vi "GenSignal.vi"(0 "Offset":dbl min=-1.0 max=1.0 step=0.1 format="%.2p", 1 "Reset Signal":bool, 2 "Formula":string="a*cos(w*t+p)", 4 "Amplitude":dbl=1.0 min=0.0 max=1.0 step=0.01 format="%.2f", 6 "Sampling Rate (MHz)":u32=1000, 7 "Phase":dbl format="%.2p", 8 "Start Time":dbl format="%#.6g", 9 "Duration (us)":dbl=1.0, 10 "Frequency (MHz)":dbl=200.0 min=0.0 max=1000.0 step=1.0 format="%#.6g", 11 "Signal Type":u16(ring) items=["Sine", "Formula"]) -> (3 "Wave":dbl[](array[numeric]), 5 "Number of points":u32)   [LabVIEW 2014]
uses:
  <vilib>/measure/NI_MAPro.lvlib
  <vilib>/measure/NI_MABase.lvlib
  <vilib>/gmath/NI_Gmath.lvlib
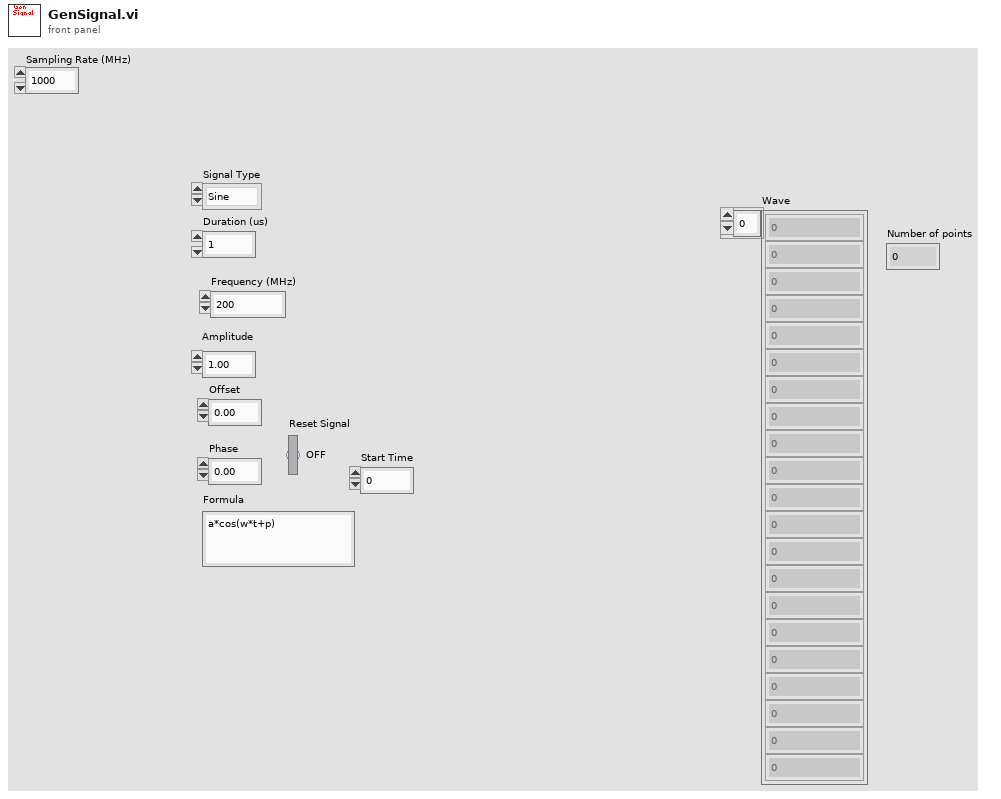
[diagram p1: front panel]
types:
  T1 = cluster{"parameter name":string, "parameter content":string}[]
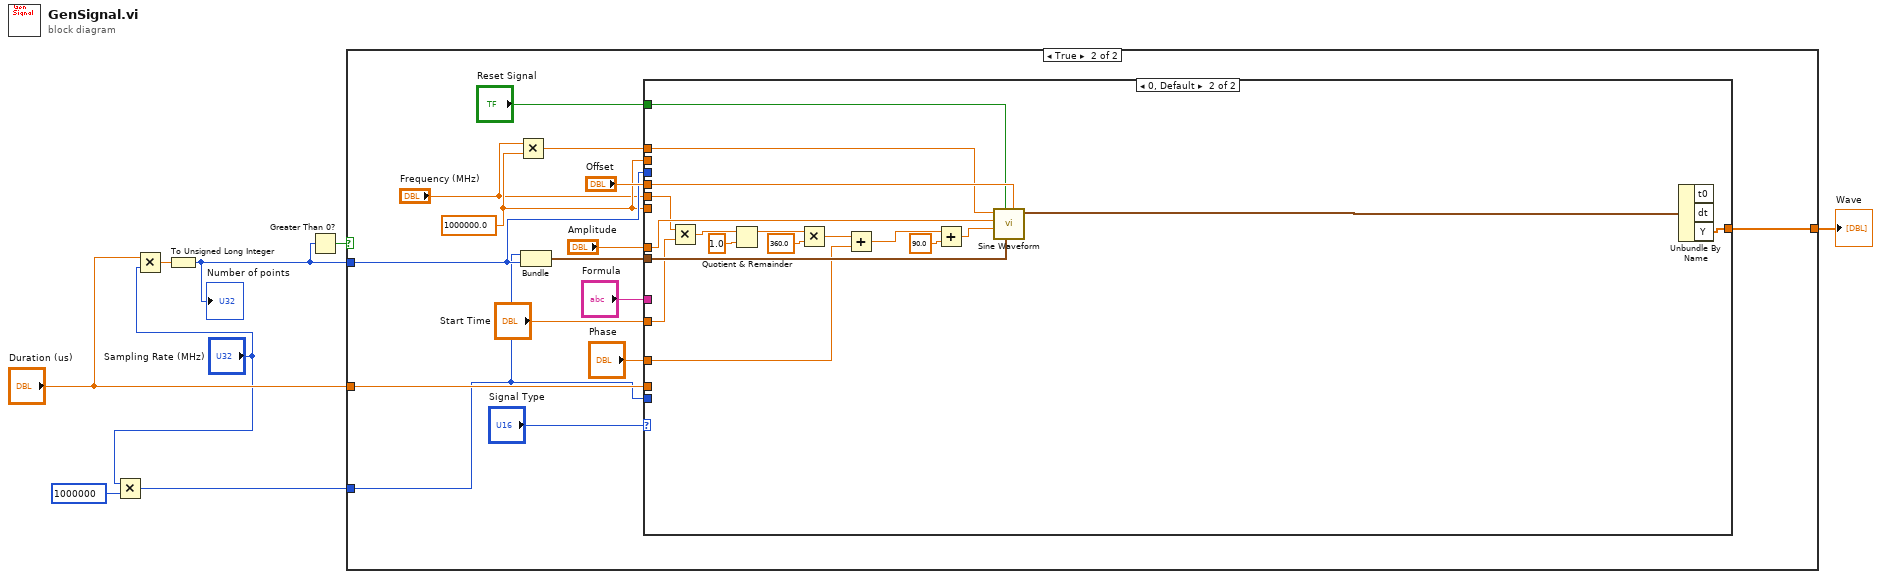
[diagram p0: block diagram]
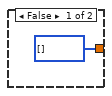
[diagram p2: hidden frame]
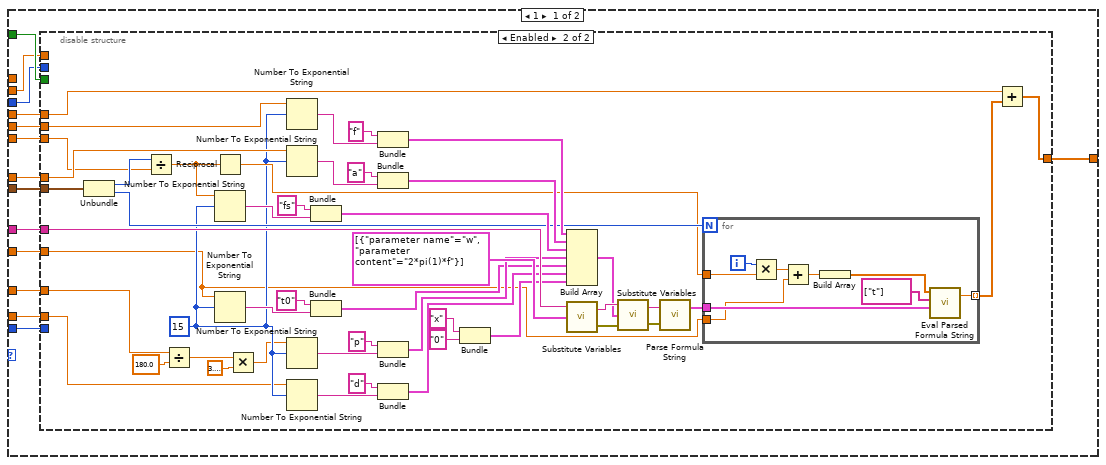
[diagram p3: hidden frame]
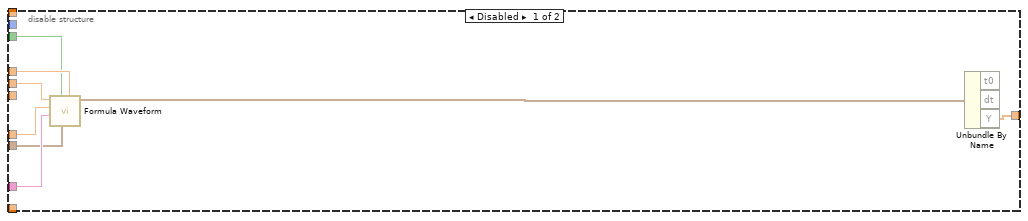
[diagram p4: hidden frame]
diagram:
  n1 = Multiply(x="Sampling Rate (MHz)", y=u32 1000000) -> (x*y=w2:u32)
  n2 = Multiply(x="Duration (us)", y="Sampling Rate (MHz)") -> (x*y=w7:dbl)
  n3 = To Unsigned Long Integer(number=w7) -> (unsigned 32bit integer=w5:u32)
  "Number of points" <- w5
  n4 = Greater Than 0?(x=w5) -> (x > 0?=w4:bool)
  n5 = case shown="True" w4 {
    tunnel: [u16[] [] w11] -> w8
    tunnel: w5 -> [_ w15]
    tunnel: "Duration (us)" -> [_ w14]
    tunnel: w2 -> [_ w10]
    frame False {
    }
    frame True {
      w13 = 1000000.0 ("y")
      n6 = Multiply(x="Frequency (MHz)", y=w13) -> (x*y=w20:dbl)
      n7 = Bundle(w10, w15) -> (w23:cluster{u32, u32})  [unwired: 1 in]
      n8 = case shown="0, Default" "Signal Type" {
        tunnel: "Offset" -> [w37 w121]
        tunnel: w23 -> [w34 w120]
        tunnel: [w35 w115] -> w11
        tunnel: "Amplitude" -> [w38 w119]
        tunnel: "Phase" -> [w30 w111]
        tunnel: w20 -> [_ w118]
        tunnel: "Formula" -> [w36 _]
        tunnel: "Reset Signal" -> [w33 w117]
        tunnel: "Start Time" -> [w32 w112]
        tunnel: w10 -> [w31 _]
        tunnel: w15 -> [w29 _]
        tunnel: w13 -> [w28 _]
        tunnel: w14 -> [w27 _]
        tunnel: "Frequency (MHz)" -> [w26 w107]
        tunnel: w13 -> [w25 _]
        frame 1 {
          n9 = disable-structure shown="Enabled" {
            disable-tunnel: w26 -> [w46 w89]
            disable-tunnel: w38 -> [w45 w88]
            disable-tunnel: w37 -> [w44 w65]
            disable-tunnel: w36 -> [w43 w94]
            disable-tunnel: [w39 w64] -> w35
            disable-tunnel: w34 -> [w42 w71]
            disable-tunnel: w33 -> [w41 _]
            disable-tunnel: w32 -> [_ w47]
            disable-tunnel: w31 -> [_ _]
            disable-tunnel: w30 -> [_ w56]
            disable-tunnel: w29 -> [_ _]
            disable-tunnel: w28 -> [_ _]
            disable-tunnel: w27 -> [_ w51]
            disable-tunnel: w25 -> [_ w48]
            frame Disabled {
              n10 = call <vilib>:"Formula Waveform.vi"("offset"=w44, "sampling info"=w42, "reset signal"=w41, "formula"=w43, "amplitude"=w45, "frequency"=w46) -> ("signal out"=w40:waveform(dbl))  [unwired: 4 in, 1 out]
              n11 = Unbundle By Name(w40) -> ("Y"=w39:dbl[])  [unwired: 2 out]
            }
            frame Enabled {
              w62 = i16 15 ("width (-)")
              n12 = Unbundle(w71) -> (w49:u32, w70:u32)
              n13 = Divide(x=w49, y=w48) -> (x/y=w50:dbl)
              n14 = Divide(x=w56, y=180.0) -> (x/y=w54:dbl)
              n15 = Reciprocal(x=w50) -> (1/x=w67:dbl)
              n16 = Number To Exponential String(number=w50, 3:w62) -> (E-format string=w80:string)  [unwired: 2 in]
              n17 = Number To Exponential String(number=w47, 3:w62) -> (E-format string=w73:string)  [unwired: 2 in]
              n18 = Multiply(x=w54, y=3.141592653589793) -> (x*y=w52:dbl)
              n19 = Number To Exponential String(number=w89, 3:w62) -> (E-format string=w86:string)  [unwired: 2 in]
              n20 = Number To Exponential String(number=w88, 3:w62) -> (E-format string=w83:string)  [unwired: 2 in]
              n21 = Number To Exponential String(number=w52, 3:w62) -> (E-format string=w76:string)  [unwired: 2 in]
              n22 = Number To Exponential String(number=w51, 3:w62) -> (E-format string=w61:string)  [unwired: 2 in]
              n23 = Bundle("fs", w80) -> (w79:cluster{string, string})  [unwired: 1 in]
              n24 = Bundle("t0", w73) -> (w72:cluster{string, string})  [unwired: 1 in]
              n25 = Bundle("f", w86) -> (w85:cluster{string, string})  [unwired: 1 in]
              n26 = Bundle("a", w83) -> (w82:cluster{string, string})  [unwired: 1 in]
              n27 = Bundle("p", w76) -> (w75:cluster{string, string})  [unwired: 1 in]
              n28 = Bundle("d", w61) -> (w60:cluster{string, string})  [unwired: 1 in]
              n29 = Bundle("x", "0") -> (w57:cluster{string, string})  [unwired: 1 in]
              n30 = Build Array(w85, w82, w79, w75, w72, w60, w57) -> (w78:cluster{string, string}[])
              n31 = call <vilib>:"Substitute Variables.vi"("Substitution Rules"=T1 [{"parameter name"="w", "parameter content"="2*pi(1)*f"}], "original formula"=w94) -> ("error out"=w68:errorcluster, "formula after substitution"=w91:string)  [unwired: 1 in]
              n32 = call <vilib>:"Substitute Variables.vi"("error in (no error)"=w68, "Substitution Rules"=w78, "original formula"=w91) -> ("error out"=w69:errorcluster, "formula after substitution"=w90:string)
              n33 = call <vilib>:"Parse Formula String.vi"("error in (no error)"=w69, "formula"=w90) -> ("Parsed Formula"=w93:cluster{"Table":i32[][], "Y Values":dbl[]})  [unwired: 1 out]
              n34 = for {
                N: w70 -> [_]
                tunnel: [w103] -> w66 mode=indexing
                tunnel: w93 -> [w102]
                tunnel: w67 -> [w100]
                tunnel: w47 -> [w96]
                i -> [w101]
                n35 = Multiply(x=w101, y=w100) -> (x*y=w97:dbl)
                n36 = Add(x=w97, y=w96) -> (x+y=w95:dbl)
                n37 = Build Array(w95) -> (w99:dbl[])
                n38 = call <vilib>:"Eval Parsed Formula String.vi"("Parsed Formula"=w102, "Variables"=string[] ["t"], "X Values"=w99) -> ("y value"=w103:dbl)  [unwired: 1 in, 1 out]
              }
              n39 = Add(x=w65, y=w66) -> (x+y=w64:dbl[])
            }
          }
        }
        frame 0, Default {
          n40 = Multiply(x=w107, y=w112) -> (x*y=w109:dbl)
          n41 = Quotient & Remainder(x=w109, y=1.0) -> (x-y*floor(x/y)=w106:dbl)  [unwired: 1 out]
          n42 = Multiply(x=w106, y=360.0) -> (x*y=w104:dbl)
          n43 = Add(x=w104, y=w111) -> (x+y=w110:dbl)
          n44 = Add(x=w110, y=90.0) -> (x+y=w114:dbl)
          n45 = call <vilib>:"Sine Waveform.vi"("offset"=w121, "sampling info"=w120, "reset signal"=w117, "phase"=w114, "amplitude"=w119, "frequency"=w118) -> ("signal out"=w116:waveform(dbl))  [unwired: 4 in, 1 out]
          n46 = Unbundle By Name(w116) -> ("Y"=w115:dbl[])  [unwired: 2 out]
        }
      }
    }
  }
  "Wave" <- w8
